vi "RX Image (SubVI).vi"(9 "columns":i32=240, 10 "rows":i32=291, 11 "Demod Bits":i8[](array[numeric])=array[633600 elements]) -> (3 "final_image":u8[][](array[numeric]))   [LabVIEW 2015]
uses:
  <vilib>/imath/engines/lvmath2/RunTimeEngine/BuiltInFunctions/zeros/NIMS_M=zeros(I32,I32).vi
  <vilib>/imathl/engines/lvmath/Functions/Error Handling/Create Error.vi
  <vilib>/imath/engines/lvmath2/RunTimeEngine/RangeToken/NIMS_Range_R2 - Integer.vi
  <instcachedir>/0/NIMS_Range_R2 - Integer_396D5D4FB869421F9245109A0975AD54.lvgen/NIMS_Range_R2 - Integer_396D5D4FB869421F9245109A0975AD54_000.vi
  <vilib>/imath/engines/lvmath2/RunTimeEngine/CommandStatement/MC_CommandStatement_break.vi
  <vilib>/imath/engines/lvmath2/RunTimeEngine/IndexRead/NIMS M(S,S).vi
  <instcachedir>/0/NIMS M(S,S)_AC51E74150A542F7991B9634C66F3096.lvgen/NIMS M(S,S)_AC51E74150A542F7991B9634C66F3096_002.vi
  <vilib>/imath/engines/lvmath2/RunTimeEngine/IndexReplace/NIMS M(S,S)=S.vi
  <instcachedir>/0/NIMS M(S,S)=S_72298AC072A24B679F5E0C14DB2DD503.lvgen/NIMS M(S,S)=S_72298AC072A24B679F5E0C14DB2DD503_002.vi
  <vilib>/imath/engines/lvmath2/RunTimeEngine/ErrorHandling/NIMS_Create Error From Enums.vi
  <vilib>/imath/engines/lvmath2/RunTimeEngine/BuiltInFunctions/uint8/NIMS_uint8(int).vi
  <instcachedir>/0/NIMS_uint8(int)_9D6EF81F86254677BB00410F9E5C6A1D.lvgen/NIMS_uint8(int)_9D6EF81F86254677BB00410F9E5C6A1D_000.vi
  <vilib>/imath/engines/lvmath2/RunTimeEngine/NodeEndStatement/NIMS_NodeEndStatement_Output.vi
  <instcachedir>/0/NIMS_NodeEndStatement_Output_53EC0D466D134D7ABD903AC30B43404B.lvgen/NIMS_NodeEndStatement_Output_53EC0D466D134D7ABD903AC30B43404B_011.vi
  <vilib>/imath/engines/lvmath2/RunTimeEngine/ErrorHandling/NIMS_Finalize Error.vi
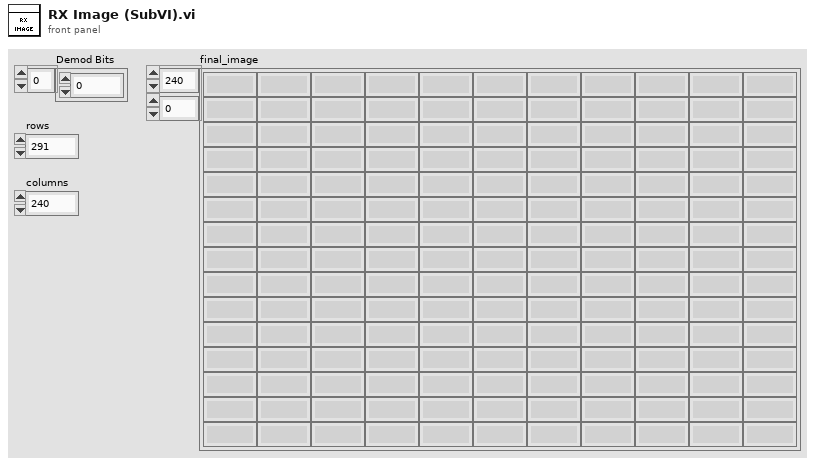
[diagram p1: front panel]
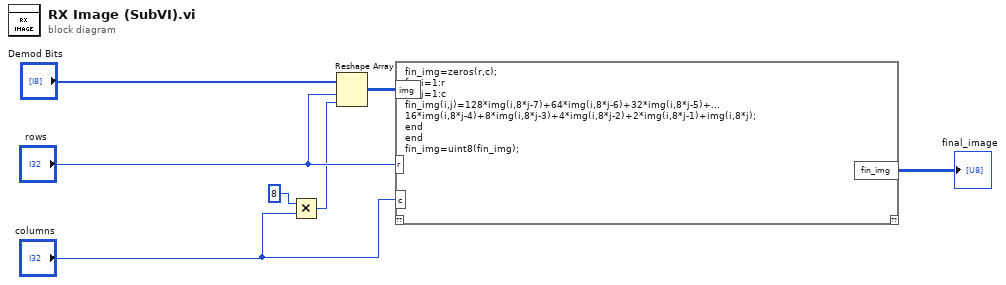
[diagram p0: block diagram]
diagram:
  n1 = Multiply(x=8, y="columns") -> (x*y=w2:i32)
  n2 = Reshape Array("Demod Bits", "rows", w2) -> (w4:i8[][])
  n3 = mathscript code="fin_img=zeros(r,c);\nfor i=1:r\nfor j=1:c\nfin_img(i,j)=128*img(i,8*j-7)+64*img(i,8*j-6)+32*img(i,8*j-5)+...\n16*img(i,8*j-4)+8*img(i,8*j-3)+4*img(i,8*j-2)+2*img(i,8*j-1)+img(i,8*j);\nend\nend\nfin_img=uint8(fin_img);"("r"="rows", "c"="columns", "img"=w4) -> ("fin_img"=→"final_image":u8[][])  [unwired: 1 in, 1 out]
